vi "asyncAcq_occurenceRef_timeStamp_viServer.vi"(0 "reference":refnum<class "OSA.lvclass">, 5 "error in (no error)":errorcluster) -> (14 "reference out":refnum<class "OSA.lvclass">, 15 "new spectrum":bool, 17 "new interferogram":bool, 19 "error out":errorcluster)   [LabVIEW 2010, in "OSA.lvclass"]
doc: "SubVI to a <B>Thorlabs_OSA_64</B> object.\n\n[GOOP 1.0]"
uses:
  OSA.lvclass
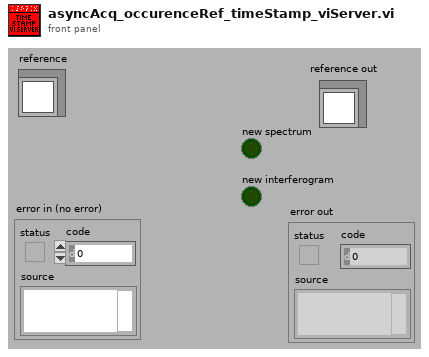
[diagram p1: front panel]
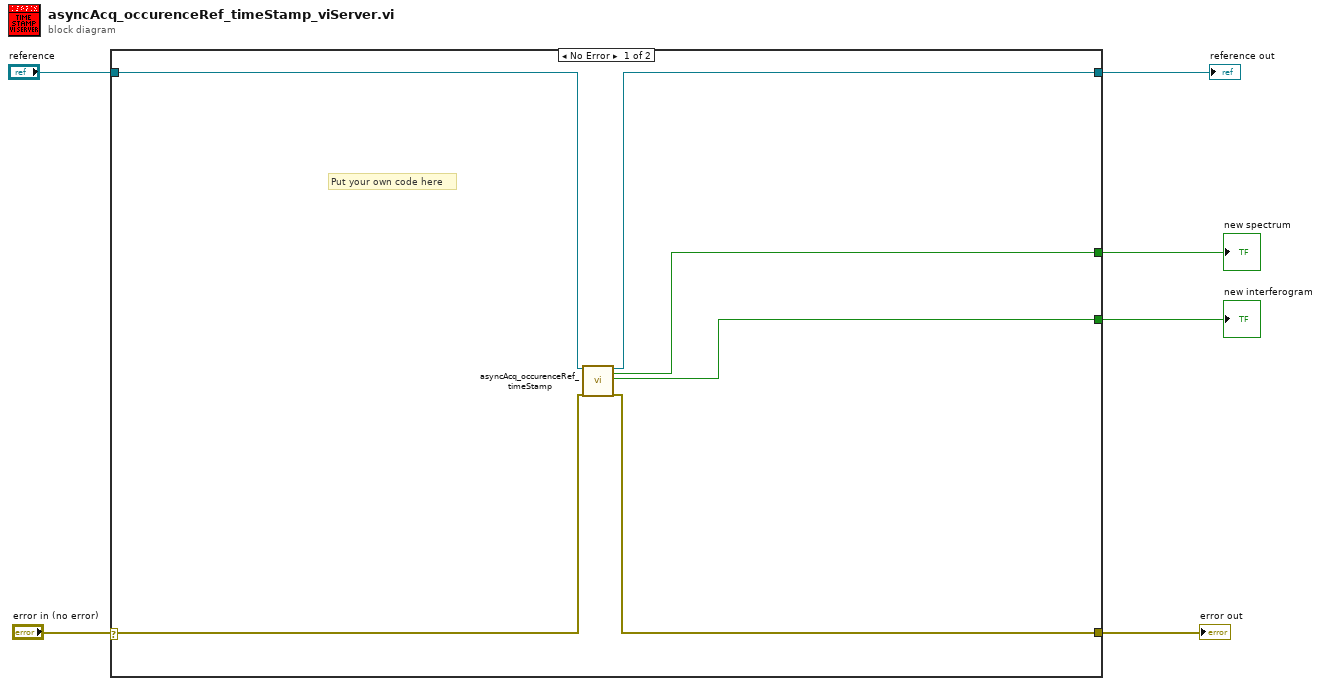
[diagram p0: block diagram]
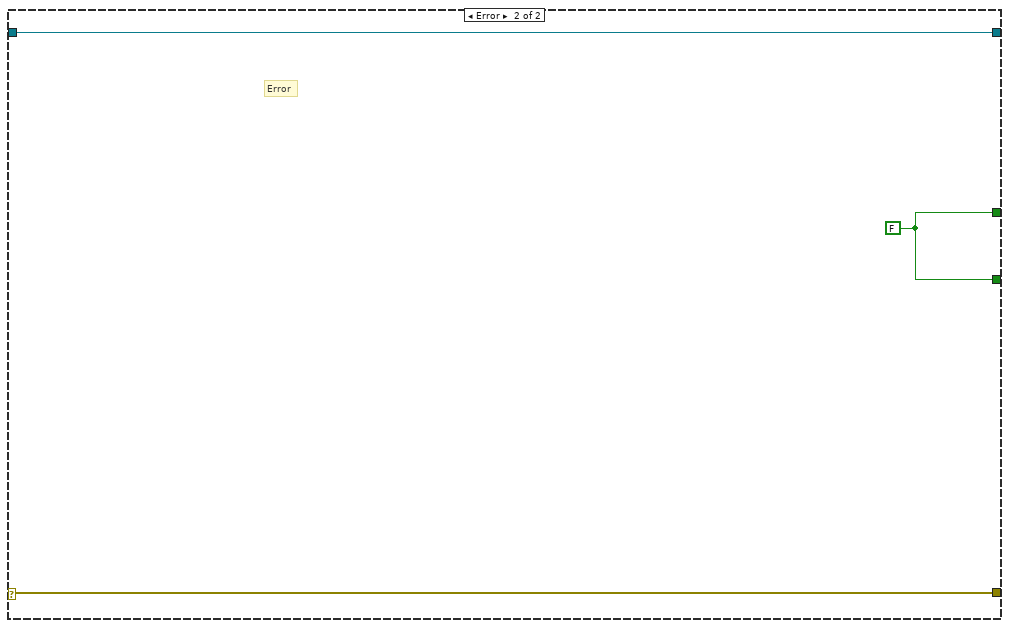
[diagram p2: hidden frame]
diagram:
  n1 = case shown="No Error" "error in (no error)" {
    selector: "error in (no error)" -> [w12 w15]
    tunnel: [w11 w15] -> w6
    tunnel: "reference" -> [w7 w13]
    tunnel: [w10 w13] -> w3
    tunnel: [w9 w14] -> w2
    tunnel: [w8 w14] -> w1
    frame No Error {
      # "Put your own code here"
      n2 = call-dynamic "asyncAcq_occurenceRef_timeStamp.vi"("reference"=w7, "error in (no error)"=w12) -> ("duplicate reference"=w10:refnum<class "OSA.lvclass">, "new spectrum"=w9:bool, "new interferogram"=w8:bool, "error out"=w11:errorcluster)  [unwired: 13 in, 1 out]
    }
    frame Error {
      w14 = FALSE ("new spectrum")
      # "Error"
    }
  }
  "error out" <- w6
  "reference out" <- w3
  "new spectrum" <- w2
  "new interferogram" <- w1
